vi "Measure_Pump.vi"(8 "error in (no error)":errorcluster, 10 "Parameters":string, 11 "reference in":refnum<class "Test_Flux_Capacitor.lvclass">) -> (0 "error out":errorcluster, 2 "Result":dbl, 3 "reference out":refnum<class "Test_Flux_Capacitor.lvclass">)   [LabVIEW 2022 SP3, in "Test_Flux_Capacitor.lvlib" / "Test_Flux_Capacitor.lvclass"]
uses:
  Test_Flux_Capacitor.lvclass
  Components/SwitchBase.lvlibp/SwitchBase.lvclass
  <vilib>/JDP Science/JSONtext/JSONtext.lvlib
panel:
  in  "Parameter_Type":T1={"Pump"=1, "Wait (msec)"=0, "Speed"=0, "State"=FALSE}
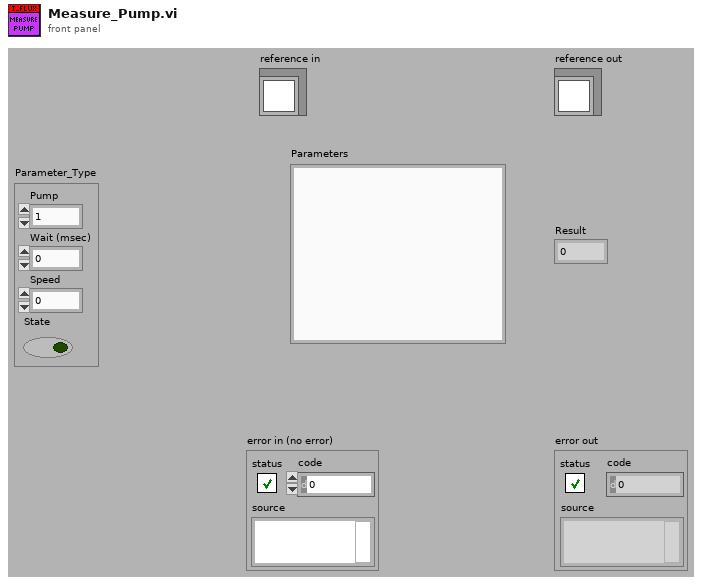
[diagram p1: front panel]
types:
  T1 = cluster{"Pump":i32, "Wait (msec)":u32, "Speed":u16, "State":bool}
  T2 = typedef "Test_Flux_Capacitor.lvlib/Test_Flux_Capacitor.lvclass/ObjectAttributes.ctl" = cluster{"Config":T3, "DMM":refnum<class "DMM_Keysight_34980A.lvclass">, "LCR":refnum<class "LCR_BK891.lvclass">, "PSU":refnum<class "PSU_Base.lvclass">, "Switch_Manager":refnum<class "SwitchBase.lvclass">, "FRAM":string, "Flux_Capacitor":refnum<class "Flux_Capacitor.lvclass">, "Frequency_Counter":refnum<class "Frequency_Counter_Base.lvclass">, "JTAG":refnum<class "JTAG_Base.lvclass">}
  T3 = typedef "Test_Flux_Capacitor.lvlib/Test_Flux_Capacitor.lvclass/Config.ctl" = cluster{"default":string}
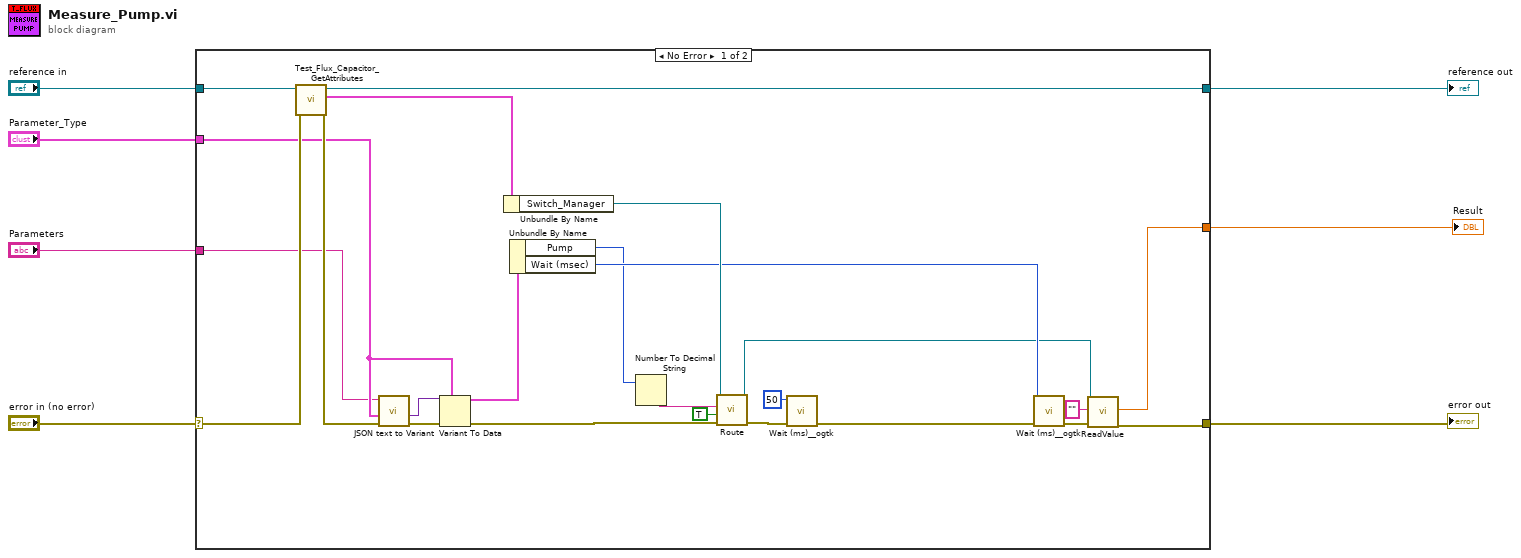
[diagram p0: block diagram]
diagram:
  n1 = case shown="No Error" "error in (no error)" {
    selector: "error in (no error)" -> [w27 w33]
    tunnel: [w29 w33] -> w6
    tunnel: [w30 w32] -> w4
    tunnel: "reference in" -> [w31 w32]
    tunnel: "Parameters" -> [w24 _]
    tunnel: "Parameter_Type" -> [w25 _]
    tunnel: [w28 _] -> w1
    frame No Error {
      n2 = call "Test_Flux_Capacitor_GetAttributes.vi"("error in (no error)"=w27, "reference in"=w31) -> ("error out"=w26:errorcluster, "Data"=w9:T2, "reference out"=w30:refnum<class "Test_Flux_Capacitor.lvclass">)  [unwired: 6 in, 1 out]
      n3 = call <vilib>:"JSON text to Variant.vi"("error in (no error)"=w26, "Data Type"=w25, "JSON"=w24) -> ("error out"=w12:errorcluster, "Variant out"=w11:variant)  [unwired: 7 in]
      n4 = Variant To Data(error in=w12, type=w25, Variant=w11) -> (data=w23:T1, error out=w14:errorcluster)
      n5 = Unbundle By Name(w9) -> ("Switch_Manager"=w22:refnum<class "SwitchBase.lvclass">)
      n6 = Unbundle By Name(w23) -> ("Pump"=w17:i32, "Wait (msec)"=w21:u32)
      n7 = Number To Decimal String(number=w17) -> (decimal integer string=w18:string)  [unwired: 1 in]
      n8 = call-dynamic "Route.vi"("error in (no error)"=w14, "Connect"=TRUE, "channel 1"=w18, "reference in"=w22) -> ("error out"=w20:errorcluster, "reference in"=w15:refnum<class "SwitchBase.lvclass">)  [unwired: 6 in]
      n9 = call <userlib>:"Wait (ms)__ogtk.vi"("error in (no error)"=w20, "milliseconds to wait"=u32 50) -> ("error out"=w8:errorcluster)  [unwired: 8 in, 1 out]
      n10 = call <userlib>:"Wait (ms)__ogtk.vi"("error in (no error)"=w8, "milliseconds to wait"=w21) -> ("error out"=w16:errorcluster)  [unwired: 8 in, 1 out]
      n11 = call-dynamic "ReadValue.vi"("reference in"=w15, "Name"="", "error in (no error)"=w16) -> ("Value"=w28:dbl, "error out"=w29:errorcluster)  [unwired: 14 in, 1 out]
    }
    frame Error {
    }
  }
  "Result" <- w1
  "error out" <- w6
  "reference out" <- w4
